vi "Configure TS Panel.vi"(8 "error in":errorcluster, 11 "HTS Test Stand in":refnum<class "HTS Test Stand.lvclass">) -> (0 "error out":errorcluster, 3 "HTS Test Stand out":refnum<class "HTS Test Stand.lvclass">)   [LabVIEW 2019, in "Test Stands.lvlib" / "HTS Test Stand.lvclass"]
uses:
  HTS Test Stand.lvclass
  Generic Test Stand/Generic Test Stand.lvclass
  C:/Users/krio/Documents/LV_Projects/test-stand/App/Generic Test Stand/Generic Test Stand.lvclass
  Results/HTS Results/HTS Results.lvclass
  Results/HTS Results/HTS Front Panel.vi
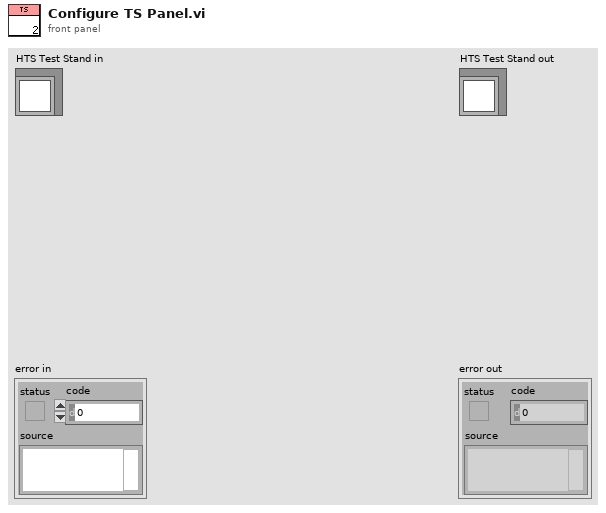
[diagram p1: front panel]
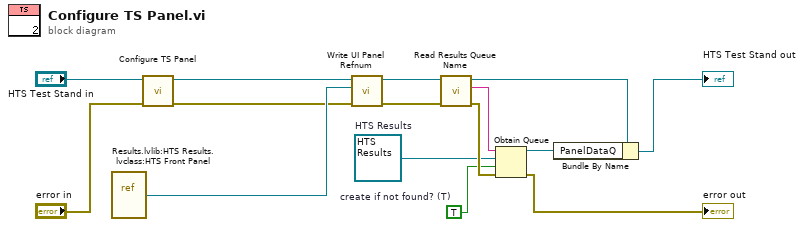
[diagram p0: block diagram]
diagram:
  w1 = refnum<class "HTS Results.lvclass"> refnum  # HTS Results
  w4 = TRUE  # create if not found? (T)
  n1 = vi-ref "Results.lvlib:HTS Results.lvclass:HTS Front Panel.vi"() -> (w15:refnum<vi>)
  n2 = call-parent "Configure TS Panel.vi"("error in (no error)"="error in", "Generic Test Stand in"="HTS Test Stand in") -> ("error out"=w11:errorcluster, "Generic Test Stand out"=w13:refnum<class "HTS Test Stand.lvclass">)  [unwired: 8 in]
  n3 = call "Write UI Panel Refnum.vi"("error in (no error)"=w11, "UI Panel Refnum"=w15, "Generic Test Stand in"=w13) -> ("error out"=w7:errorcluster, "Generic Test Stand out"=w10:refnum<class "HTS Test Stand.lvclass">)  [unwired: 7 in]
  n4 = call "Read Results Queue Name.vi"("error in (no error)"=w7, "Generic Test Stand in"=w10) -> ("error out"=w5:errorcluster, "Results Queue Name"=w6:string, "Generic Test Stand out"=w9:refnum<class "HTS Test Stand.lvclass">)  [unwired: 7 in]
  n5 = Obtain Queue(name (unnamed)=w6, element data type=w1, create if not found? (T)=w4, error in (no error)=w5) -> (queue out=w3:refnum<queue>, error out=→"error out":errorcluster)  [unwired: 1 in, 1 out]
  n6 = Bundle By Name(cluster=w9, "PanelDataQ"=w3) -> (→"HTS Test Stand out":refnum<class "HTS Test Stand.lvclass">)
